vi "TDMSAdv close.vi"(8 "error in (no error)":errorcluster, 11 "TDMSAdv in":refnum<class "TDMSAdv.lvclass">) -> (0 "error out":errorcluster, 2 "filePath":path, 3 "TDMSAdv out":refnum<class "TDMSAdv.lvclass">)   [LabVIEW 2018, in "TDMSAdv.lvclass"]
uses:
  TDMSAdv.lvclass
  TDMSAdv.lvclass/TDMSAdv.ctl
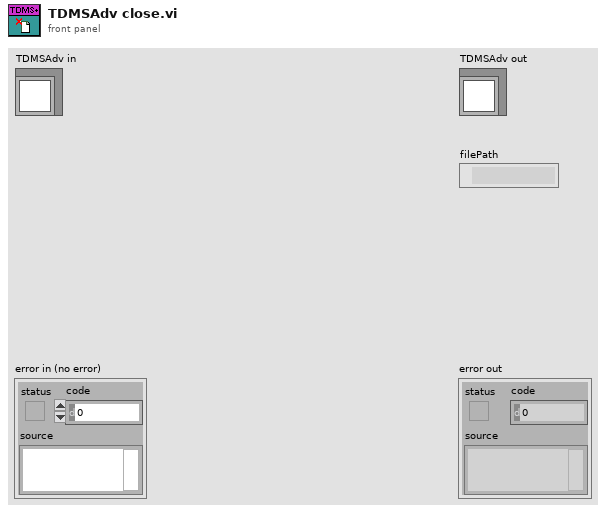
[diagram p1: front panel]
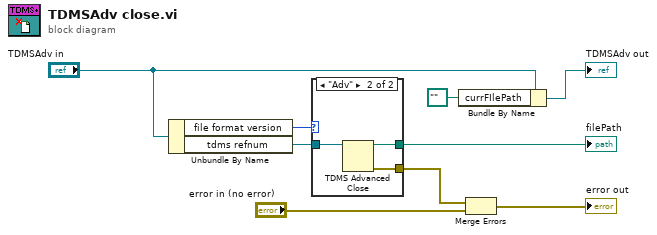
[diagram p0: block diagram]
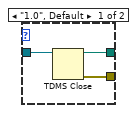
[diagram p2: hidden frame]
diagram:
  n1 = Unbundle By Name("TDMSAdv in") -> ("file format version"=w5:enum16{"1.0", "2.0", "Adv"}, "tdms refnum"=w6:refnum<k34>)
  n2 = case shown="\"Adv\"" w5 {
    tunnel: [w10 w15] -> w3
    tunnel: [w11 w14] -> w7
    tunnel: w6 -> [w12 w13]
    frame "1.0", Default {
      n3 = TDMS Close(11:w12) -> (0:w10:errorcluster, 3:w11:path)  [unwired: 1 in]
    }
    frame "Adv" {
      n4 = TDMS Advanced Close(11:w13) -> (0:w15:errorcluster, 3:w14:path)  [unwired: 3 in]
    }
  }
  "filePath" <- w7
  n5 = Bundle By Name(cluster="TDMSAdv in", "currFIlePath"=path "" ("tdmsPath")) -> (→"TDMSAdv out":refnum<class "TDMSAdv.lvclass">)
  n6 = Merge Errors(w3, "error in (no error)") -> (→"error out":errorcluster)
